vi "Digital Read Pulse Width.vi"(5 "Stimulus Pulse (Active High)":T2, 6 "Timeout  (250 mS)":u32=250, 7 "Incoming Pulse Polarity (Active High)":T1=enum."Active High", 8 "Error In":errorcluster, 9 "DO Channel":u8, 10 "DI Channel":u8, 11 "LINX Resource":T3) -> (0 "Error Out":errorcluster, 2 "Pulse Width (uS)":u32, 3 "LINX Resource":T3)   [LabVIEW 2020, in "LMH-LINX.lvlib"]
doc: "Read a digital pulse width. Use the Stimulus input to specify a pulse type to send before measuring the response pulse."
uses:
  LMH-LINX.lvlib
  Private/Type Defs/LINX Ref.ctl
  Private/Type Defs/Platform.ctl
  Private/Type Defs/Interface.ctl
  Private/Device/Type Defs/LINX Device Config.ctl
  Private/Device/Type Defs/TCP Config.ctl
  Private/Device/Type Defs/Channels.ctl
  Private/Device/Type Defs/Stimulus Pulse.ctl
  Private/Device/Type Defs/Pulse Polarity.ctl
  Private/Type Defs/Peripheral.ctl
  Private/Type Defs/Error Type.ctl
  Private/Device/Device.lvlib
  Private/myRIO/myRIO.lvlib
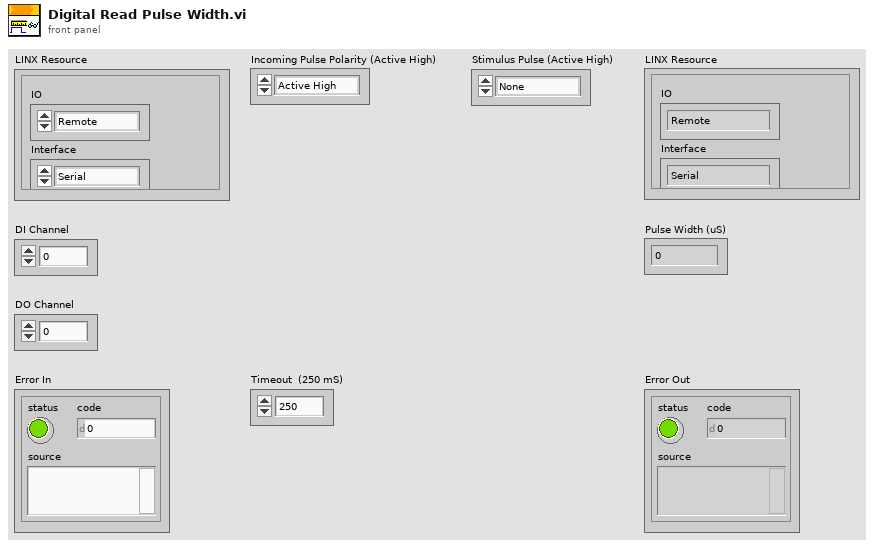
[diagram p1: front panel]
types:
  T1 = typedef "LMH-LINX.lvlib/Device.lvlib/Pulse Polarity.ctl" = enum8{"Active Low", "Active High"}
  T2 = typedef "LMH-LINX.lvlib/Device.lvlib/Stimulus Pulse.ctl" = enum16{"None", "Active Low", "Active High"}
  T3 = typedef "LMH-LINX.lvlib/LINX Ref.ctl" = cluster{"IO":T4, "Interface":T5, "LINX Device Config":T6}
  T4 = typedef "LMH-LINX.lvlib/Platform.ctl" = enum16{"Remote", "Local"}
  T5 = typedef "LMH-LINX.lvlib/Interface.ctl" = enum16{"Serial", "TCP"}
  T6 = typedef "LMH-LINX.lvlib/Device.lvlib/LINX Device Config.ctl" = cluster{"Interface":T5, "COM Port":refnum<visa-resource-name>, "TCP Configuration":T7, "Device Family":u8, "Device ID":u8, "Device Name":string, "TCP Ref":refnum<k5>, "Channels":T8}
  T7 = typedef "LMH-LINX.lvlib/Device.lvlib/TCP Config.ctl" = cluster{"IP Address":string, "Port":u16}
  T8 = typedef "LMH-LINX.lvlib/Channels.ctl" = cluster{"DI":u8[], "DO":u8[], "AI":u8[], "AO":u8[], "PWM":u8[], "QE":u8[], "UART":u8[], "I2C 2":u8[], "SPI":u8[], "CAN":u8[], "Servo":u8[], "AI Ref (V)":dbl, "AI Resolution (Bits)":u8, "AO Ref (V)":dbl, "AO Resolution (Bits)":u8}
  T9 = typedef "LMH-LINX.lvlib/Peripheral.ctl" = enum8{"DI", "DO", "AI", "AO", "PWM", "QE", "UART", "I2C", "SPI", "CAN", "Servo"}
  T10 = typedef "LMH-LINX.lvlib/Error Type.ctl" = enum16{"Unknown", "Timeout", "Corrupt Return Packet", "Unable To Connect", "Command Not Supported", "Channel DNE", "Invalid COM Config", "Firmware Version Mismatch", "myRIO Support", "CMD Specific Error", "Local IO Not Supported"}
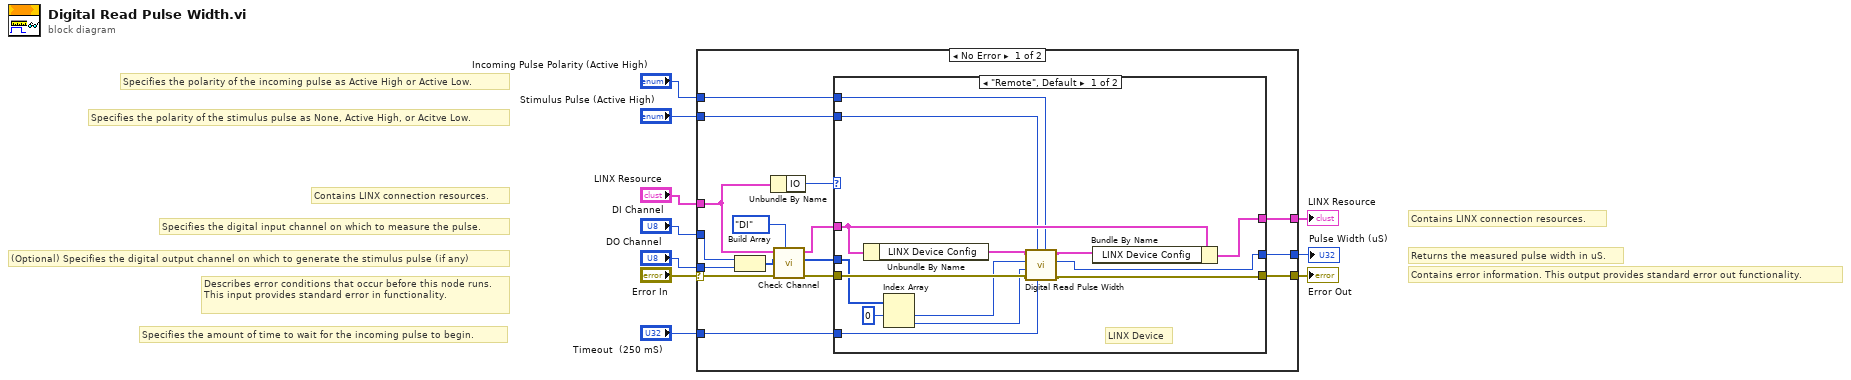
[diagram p0: block diagram]
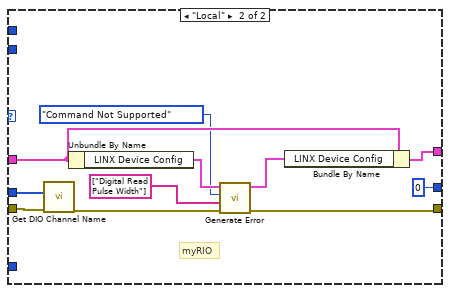
[diagram p2: hidden frame]
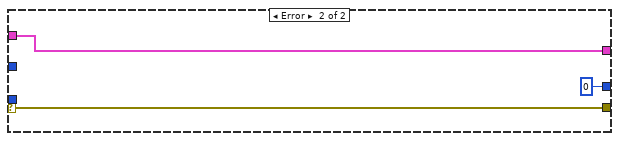
[diagram p3: hidden frame]
diagram:
  # "Returns the measured pulse width in uS."
  # "Specifies the amount of time to wait for the incoming pulse to begin."
  # "(Optional) Specifies the digital output channel on which to generate the stimulus pulse (if any)"
  # "Specifies the digital input channel on which to measure the pulse."
  # "Specifies the polarity of the stimulus pulse as None, Active High, or Acitve Low."
  # "Specifies the polarity of the incoming pulse as Active High or Active Low."
  # "Contains LINX connection resources."
  # "Contains error information. This output provides standard error out functionality."
  # "Contains LINX connection resources."
  # "Describes error conditions that occur before this node runs. This input provides standard error in functionality."
  n1 = case shown="No Error" "Error In" {
    selector: "Error In" -> [w11 w54]
    tunnel: [w25 w54] -> w10
    tunnel: [w24 w53] -> w9
    tunnel: "LINX Resource" -> [w19 w53]
    tunnel: "DI Channel" -> [w18 _]
    tunnel: [w16 u32 0 ("Pulse Width (uS)")] -> w6
    tunnel: "Incoming Pulse Polarity (Active High)" -> [w15 _]
    tunnel: "DO Channel" -> [w14 _]
    tunnel: "Stimulus Pulse (Active High)" -> [w13 _]
    tunnel: "Timeout  (250 mS)" -> [w12 _]
    frame No Error {
      n2 = Build Array(w18, w14) -> (w17:u8[])
      n3 = Unbundle By Name(w19) -> ("IO"=w26:T4)
      n4 = call "Check Channel.vi"("Peripheral"=Peripheral."DI", "Error In"=w11, "Channels"=w17, "LINX Resource"=w19) -> ("Error Out"=w23:errorcluster, "Channels"=w22:u8[], "LINX Resource"=w20:T3)  [unwired: 5 in]
      n5 = case shown="\"Remote\", Default" w26 {
        tunnel: w23 -> [w36 w51]
        tunnel: w20 -> [w40 w44]
        tunnel: [w35 w48] -> w25
        tunnel: [w39 w45] -> w24
        tunnel: w22 -> [w34 w50]
        tunnel: [w31 u32 0 ("Pulse Width (uS)")] -> w16
        tunnel: w15 -> [w29 _]
        tunnel: w13 -> [w30 _]
        tunnel: w12 -> [w28 _]
        frame "Remote", Default {
          # "LINX Device"
          n6 = Unbundle By Name(w40) -> ("LINX Device Config"=w37:T6)
          n7 = Index Array(array=w34, index #1=0 ("index")) -> (element #1=w32:u8, element #2=w27:u8)  [unwired: 1 in]
          n8 = call "Digital Read Pulse Width.vi"("Incoming Pulse Polarity (Active High)"=w29, "Timeout  (250 mS)"=w28, "Stimulus Pulse (Active High)"=w30, "Error In"=w36, "DO Channel (0)"=w27, "DI Channel (0)"=w32, "LINX Device Config"=w37) -> ("Error Out"=w35:errorcluster, "Pulse Width (uS)"=w31:u32, "LINX Device Config"=w38:T6)  [unwired: 2 in]
          n9 = Bundle By Name(cluster=w40, "LINX Device Config"=w38) -> (w39:T3)
        }
        frame "Local" {
          # "myRIO"
          n10 = call "Get DIO Channel Name.vi"("Error In"=w51, "DIO Channel Nums"=w50) -> ("Error Out"=w49:errorcluster)  [unwired: 8 in, 1 out]
          n11 = Unbundle By Name(w44) -> ("LINX Device Config"=w46:T6)
          n12 = call "Generate Error.vi"("Error In"=w49, "Arguments"=string[] ["Digital Read Pulse Width"], "Error Type"=Error_Type."Command Not Supported", "LINX Device Config"=w46) -> ("Error Out"=w48:errorcluster, "Dup LINX Device Config"=w47:T6)  [unwired: 6 in]
          n13 = Bundle By Name(cluster=w44, "LINX Device Config"=w47) -> (w45:T3)
        }
      }
    }
    frame Error {
    }
  }
  "Error Out" <- w10
  "LINX Resource" <- w9
  "Pulse Width (uS)" <- w6
